vi "responseInterval.vi"() -> ()   [LabVIEW 2014]
panel:
  out "result":bool
  out "Lick":bool
  in  "Lick":bool
  in  "index":i32
  in  "Params":T1={"Mice ID"=[], "ExpType"=[], "Trial Interval"=[], "Pulse Duration"=[158.0, 152.0, 156.0, 167.0, 172.0], "microL_per_pulse"=[6.0, 6.0, 6.0, 6.0, 6.0], "Response Interval"=[1000.0, 1000.0, 1000.0, 1000.0, 1000.0], "Bad Delay"=[], "Response Period"=[], "liquid_type"="water", "Stimuli"=[], "Rewarded Stimuli"=[]}
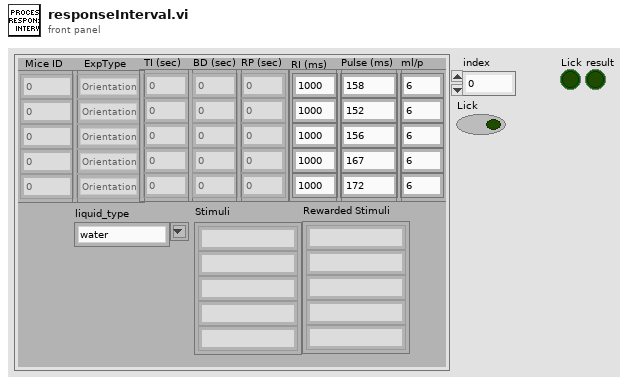
[diagram p1: front panel]
types:
  T1 = cluster{"Mice ID":dbl[], "ExpType":enum16{"Orientation", "Calibrate", "Freerun", "BW"}[], "Trial Interval":dbl[], "Pulse Duration":dbl[], "microL_per_pulse":dbl[], "Response Interval":dbl[], "Bad Delay":dbl[], "Response Period":dbl[], "liquid_type":string, "Stimuli":string[], "Rewarded Stimuli":string[]}
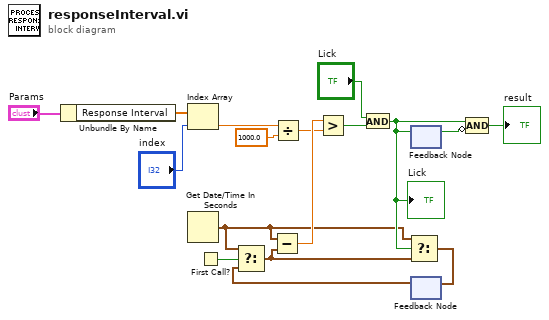
[diagram p0: block diagram]
diagram:
  n1 = Unbundle By Name("Params") -> ("Response Interval"=w11:dbl[])
  n2 = Index Array(array=w11, index="index") -> (element=w9:dbl)
  n3 = Get Date/Time In Seconds() -> (seconds since 1Jan1904=w4:timestamp)
  n4 = First Call?() -> (First Call?: T/F=w17:bool)
  n5 = Divide(x=w9, y=1000.0) -> (x/y=w13:dbl)
  n6 = feedback #1() -> (w7:bool)  [unwired: 1 in]
  n7 = feedback #2() -> (w1:timestamp)  [unwired: 1 in]
  n8 = Select(t=w4, s=w17, f=w1) -> (s? t:f=w3:timestamp)
  n9 = Subtract(x=w4, y=w3) -> (x-y=w16:dbl)
  n10 = Greater?(x=w16, y=w13) -> (0:w15:bool)
  n11 = And(x="Lick", y=w15) -> (x .and. y?=w5:bool)
  "Lick" <- w5
  n12 = Select(t=w4, s=w5, f=w3) -> (s? t:f=w2:timestamp)
  n13 = feedback-in #1(w5) -> ()
  n14 = feedback-in #2(w2) -> ()
  n15 = Compound Arithmetic op=AND(w5, invert w7) -> (→"result":bool)
